vi "Destroy Events Refs.vi"(11 "Hello World Event in":refnum<class "Hello World Event.lvclass">) -> (3 "Hello World Event out":refnum<class "Hello World Event.lvclass">)   [LabVIEW 2021, in "Hello World Event.lvlib" / "Hello World Event.lvclass"]
uses:
  Hello World Event.lvclass
  Hello World Event.lvclass/Hello World Event.ctl
  Actor/Event Actor/Event Actor.lvclass
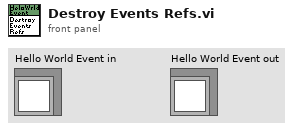
[diagram p1: front panel]
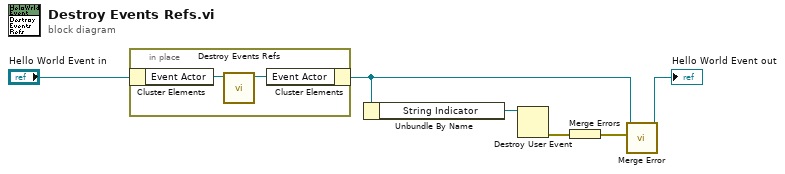
[diagram p0: block diagram]
diagram:
  n1 = in-place {
    n2 = in-place-cluster #1("Hello World Event in") -> ("Event Actor"=w8:refnum<class "Event Actor.lvclass">)
    n3 = call-dynamic "Destroy Events Refs.vi"("Event Actor in"=w8) -> ("Event Actor out"=w7:refnum<class "Event Actor.lvclass">)  [unwired: 10 in]
    n4 = in-place-cluster #1("Event Actor"=w7) -> (w1:refnum<class "Hello World Event.lvclass">)
  }
  n5 = Unbundle By Name(w1) -> ("String Indicator"=w6:refnum<user-event>)
  n6 = Destroy User Event(user event=w6) -> (error out=w5:errorcluster)  [unwired: 1 in]
  n7 = Merge Errors(w5) -> (w4:errorcluster)
  n8 = call-dynamic "Merge Error.vi"("Error"=w4, "Set Error in"=w1) -> ("Set Error out"=→"Hello World Event out":refnum<class "Hello World Event.lvclass">)  [unwired: 9 in]
